vi "Set_Plot_Names.vi"(7 "error in (no error)":errorcluster caption="entrée d'erreur (pas d'erreur)", 9 "Nom des traces":string[](array[string]), 10 "Ref au graphe":refnum<vi>) -> (0 "error out":errorcluster caption="sortie d'erreur")   [LabVIEW 2013]
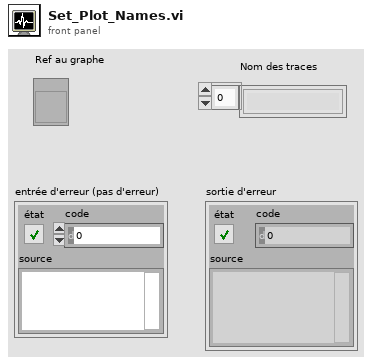
[diagram p1: front panel]
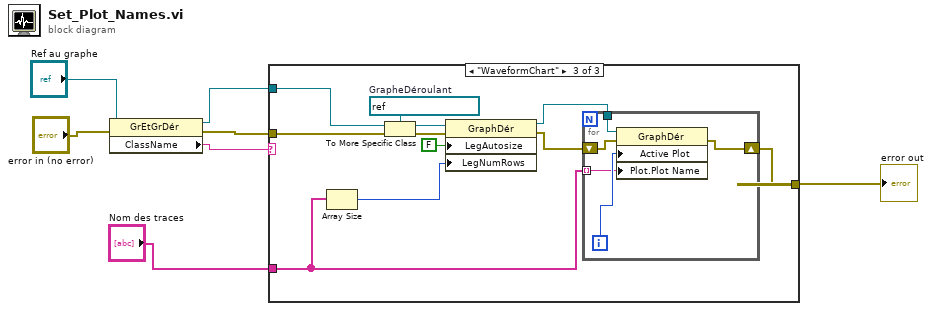
[diagram p0: block diagram]
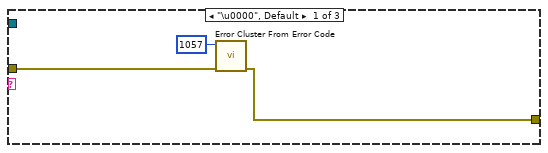
[diagram p2: hidden frame]
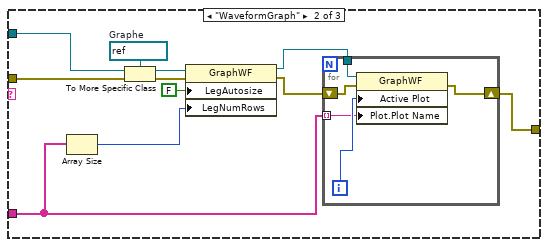
[diagram p3: hidden frame]
diagram:
  n1 = property class="GrEtGrDér"(reference="Ref au graphe", error in="error in (no error)") -> (reference out=w3:refnum<vi>, error out=w5:errorcluster, "ClassName"=w1:string)
  n2 = case shown="\"WaveformChart\"" w1 {
    tunnel: w5 -> [w9 w20 w36]
    tunnel: [w8 w12 w28] -> w4
    tunnel: w3 -> [_ w19 w35]
    tunnel: "Nom des traces" -> [_ w11 w27]
    frame "\u0000", Default {
      n3 = call <vilib>:"Error Cluster From Error Code.vi"("error in (no error)"=w9, "error code (0)"=1057) -> ("error out"=w8:errorcluster)  [unwired: 7 in]
    }
    frame "WaveformGraph" {
      w21 = refnum<vi> refnum  # Graphe
      n4 = Array Size(array=w11) -> (size(s)=w15:i32)
      n5 = To More Specific Class(target class=w21, reference=w19, error in=w20) -> (specific class reference=w16:refnum<vi>, error out=w17:errorcluster)
      n6 = property class="GraphWF"(reference=w16, error in=w17, "LegAutosize"=FALSE ("Légende:Redimensionnement automatique"), "LegNumRows"=w15) -> (reference out=w13:refnum<vi>, error out=w14:errorcluster)
      n7 = for {
        tunnel: w13 -> [w24]
        shift-right: [w23] -> w12
        shift-left: w14 -> [w25]
        tunnel: w11 -> [w22] mode=indexing
        i -> [w26]
        n8 = property class="GraphWF"(reference=w24, error in=w25, "Active Plot"=w26, "Plot.Plot Name"=w22) -> (error out=w23:errorcluster)  [unwired: 1 out]
      }
    }
    frame "WaveformChart" {
      w37 = refnum<vi> refnum  # GrapheDéroulant
      n9 = Array Size(array=w27) -> (size(s)=w31:i32)
      n10 = To More Specific Class(target class=w37, reference=w35, error in=w36) -> (specific class reference=w32:refnum<vi>, error out=w33:errorcluster)
      n11 = property class="GraphDér"(reference=w32, error in=w33, "LegAutosize"=FALSE ("Légende:Redimensionnement automatique"), "LegNumRows"=w31) -> (reference out=w29:refnum<vi>, error out=w30:errorcluster)
      n12 = for {
        tunnel: w29 -> [w40]
        shift-right: [w39] -> w28
        shift-left: w30 -> [w41]
        tunnel: w27 -> [w38] mode=indexing
        i -> [w42]
        n13 = property class="GraphDér"(reference=w40, error in=w41, "Active Plot"=w42, "Plot.Plot Name"=w38) -> (error out=w39:errorcluster)  [unwired: 1 out]
      }
    }
  }
  "error out" <- w4
